vi "Run.vi"(8 "error in (no error)":errorcluster, 11 "Save Image in":refnum<class "Save Image.lvclass">) -> (0 "error out":errorcluster, 3 "Save Image out":refnum<class "Save Image.lvclass">)   [LabVIEW 2018, in "Save Image.lvclass"]
doc: "Run the Save Image class"
uses:
  Save Image.lvclass
  Save Image.lvclass/Save Image.ctl
  Channel/Channel.lvclass/Channel.ctl
  Sim_Ixon_Ultra/Sim_Ixon_Ultra.lvclass
  C:/Users/Denis/Desktop/S4ACS/S4ACS/Sim_CCD/Sim_CCD.lvclass
  State Machine/State Machine.lvclass
  Channel/Channel.lvclass
  Sim_CCD/Sim_CCD.lvclass
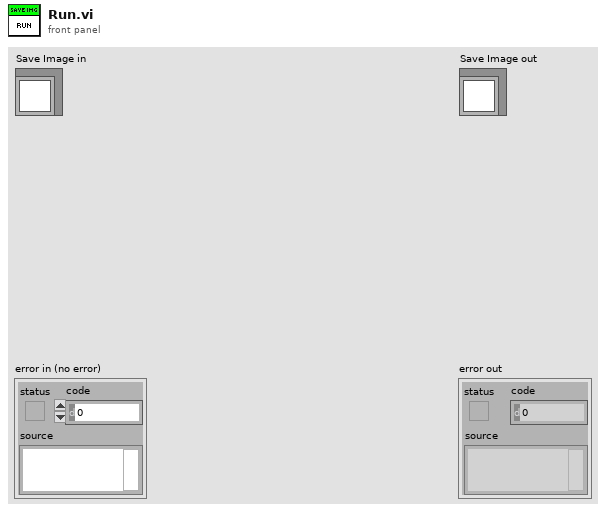
[diagram p1: front panel]
types:
  T1 = cluster{"suffix":string, "#CYCLES":u32, "#SEQS":u32, "WAVEPLATE_POS":u16, "Waveplate positions":u8[]}
  T2 = cluster{"CYCLES_DONE":u16, "LAST_IMAGE_NAME":string, "USED_DISK_SPACE":u16, "IMAGE_INDEX":u32, "SEQS_DONE":u16, "acquisition error":bool, "S4ICS comm attempts":u8}
  T3 = cluster{"FRAMES_DONE":u16, "CCD_STATUS":string, "CURRENT_TEMPERATURE":i16, "TEMPERATURE_STATUS":string, "FRAME_EXPOSURE_TIME":sgl, "SERIAL_NUMBER":u16, "ACQUIRING":bool, "POWER":bool}
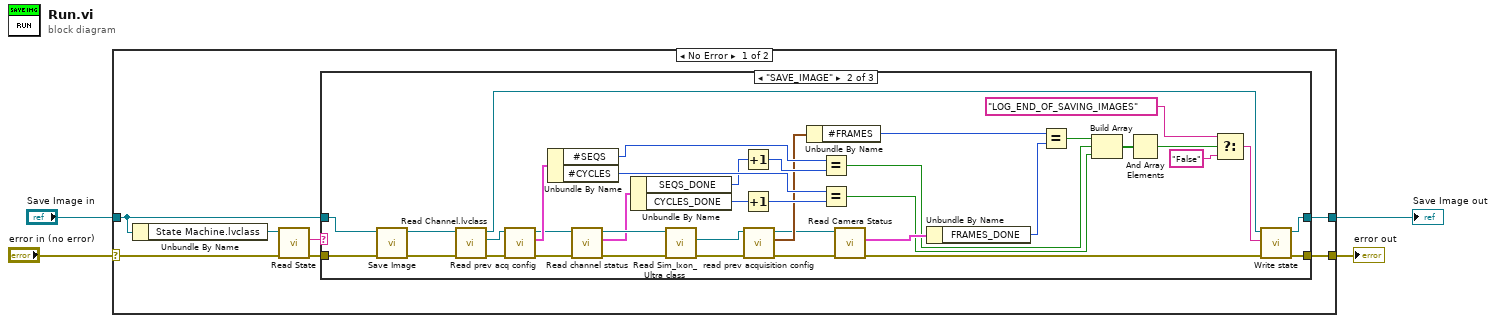
[diagram p0: block diagram]
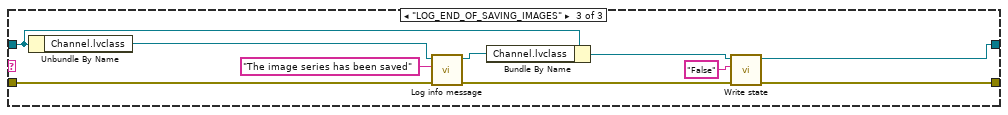
[diagram p3: hidden frame]
diagram:
  n1 = case shown="No Error" "error in (no error)" {
    selector: "error in (no error)" -> [w10 w63]
    tunnel: [w5 w63] -> w3
    tunnel: [w6 w62] -> w2
    tunnel: "Save Image in" -> [w8 w62]
    frame No Error {
      n2 = Unbundle By Name(w8) -> ("State Machine.lvclass"=w11:refnum<class "State Machine.lvclass">)
      n3 = call-dynamic "Read State.vi"("error in (no error)"=w10, "State Machine in"=w11) -> ("error out"=w7:errorcluster, "State"=w9:string)  [unwired: 7 in, 1 out]
      n4 = case shown="\"SAVE_IMAGE\"" w9 {
        tunnel: w8 -> [w13 w51 w52]
        tunnel: w7 -> [w12 w50 w55]
        tunnel: [w13 w49 w61] -> w6
        tunnel: [w12 w48 w60] -> w5
        frame "False", Default {
        }
        frame "SAVE_IMAGE" {
          n5 = call "Save Image.vi"("error in (no error)"=w50, "Save Image in"=w51) -> ("error out"=w47:errorcluster, "Save Image out"=w46:refnum<class "Save Image.lvclass">)  [unwired: 8 in]
          n6 = call-dynamic "Read Channel.lvclass.vi"("error in (no error)"=w47, "Save Image in"=w46) -> ("error out"=w29:errorcluster, "Channel.lvclass"=w30:refnum<class "Channel.lvclass">, "Save Image out"=w41:refnum<class "Save Image.lvclass">)  [unwired: 7 in]
          n7 = call-dynamic "Read prev acq config.vi"("error in (no error)"=w29, "Channel in"=w30) -> ("error out"=w20:errorcluster, "prev acq config"=w28:T1, "Channel out"=w17:refnum<class "Channel.lvclass">)  [unwired: 7 in]
          n8 = Unbundle By Name(w28) -> ("#SEQS"=w27:u32, "#CYCLES"=w26:u32)
          n9 = call-dynamic "Read channel status.vi"("error in (no error)"=w20, "Channel in"=w17) -> ("error out"=w19:errorcluster, "channel status"=w16:T2, "Channel out"=w18:refnum<class "Channel.lvclass">)  [unwired: 7 in]
          n10 = Unbundle By Name(w16) -> ("SEQS_DONE"=w15:u16, "CYCLES_DONE"=w14:u16)
          n11 = call "Read Sim_Ixon_Ultra class.vi"("error in (no error)"=w19, "Channel in"=w18) -> ("error out"=w22:errorcluster, "Sim_Ixon_Ultra.lvclass"=w21:refnum<class "Sim_Ixon_Ultra.lvclass">)  [unwired: 7 in, 1 out]
          n12 = Increment(x=w15) -> (x+1=w37:u16)
          n13 = Increment(x=w14) -> (x+1=w36:u16)
          n14 = call "read prev acquisition config.vi"("error in (no error)"=w22, "Simulated_CCD_Camera in"=w21) -> ("error out"=w23:errorcluster, "Prev SET parameters"=w25:cluster{"EXPTIME":dbl, "#FRAMES":u32}, "Simulated_CCD_Camera out"=w24:refnum<class "Sim_Ixon_Ultra.lvclass">)  [unwired: 7 in]
          n15 = Unbundle By Name(w25) -> ("#FRAMES"=w38:u32)
          n16 = Equal?(x=w27, y=w37) -> (x = y?=w34:bool)
          n17 = Equal?(x=w26, y=w36) -> (x = y?=w35:bool)
          n18 = call "Read Camera Status.vi"("error in (no error)"=w23, "CCDCamera in"=w24) -> ("error out"=w40:errorcluster, "camera status"=w45:T3)  [unwired: 7 in, 1 out]
          n19 = Unbundle By Name(w45) -> ("FRAMES_DONE"=w39:u16)
          n20 = Equal?(x=w38, y=w39) -> (x = y?=w33:bool)
          n21 = Build Array(w33, w34, w35) -> (w32:bool[])
          n22 = And Array Elements(Boolean array=w32) -> (logical AND=w31:bool)
          n23 = Select(t="LOG_END_OF_SAVING_IMAGES" ("String"), s=w31, f="False" ("String")) -> (s? t:f=w42:string)
          n24 = call "Write state.vi"("error in (no error)"=w40, "String"=w42, "Save Image in"=w41) -> ("error out"=w48:errorcluster, "Save Image out"=w49:refnum<class "Save Image.lvclass">)  [unwired: 7 in]
        }
        frame "LOG_END_OF_SAVING_IMAGES" {
          n25 = Unbundle By Name(w52) -> ("Channel.lvclass"=w58:refnum<class "Channel.lvclass">)
          n26 = call "Log info message.vi"("error in (no error)"=w55, "String"="The image series has been saved", "Channel in"=w58) -> ("error out"=w54:errorcluster, "Channel out"=w57:refnum<class "Channel.lvclass">)  [unwired: 7 in]
          n27 = Bundle By Name(cluster=w52, "Channel.lvclass"=w57) -> (w53:refnum<class "Save Image.lvclass">)
          n28 = call "Write state.vi"("error in (no error)"=w54, "String"="False", "Save Image in"=w53) -> ("error out"=w60:errorcluster, "Save Image out"=w61:refnum<class "Save Image.lvclass">)  [unwired: 7 in]
        }
      }
    }
    frame Error {
    }
  }
  "error out" <- w3
  "Save Image out" <- w2
